vi "5.3-4.7.3-What Client.vi"() -> ()   [LabVIEW 2010]
doc: "This VI implements a client for the Named Service UDP Server.vi.\nIt connects to a service by specifying the server address and the name of the service. After sending a 'Hello' string to the server, the client receives the string sent by the server, displays the string and closes the connection.\n\n<b>Note:</b> This VI is built to work with the Named Service UDP Server.vi in UDP.llb."
uses:
  5.0-Global.vi
  <vilib>/addons/internet/NI_InternetTK_Common_VIs.lvlib
  <vilib>/Utility/tcp.llb/UDP Multicast Open.vi
  3-Midbrain/3.3-What/_typedefs/3.3.1-LIDAR Data Typedef.ctl
  4-High Neurons/4.3-What Sensor Typedef.ctl
  4-High Neurons/4.0-Timing Badass.ctl
panel:
  out "Super Heart Beat":T1
  out "data":T2
  out "Error":errorcluster
  in  "stop":bool
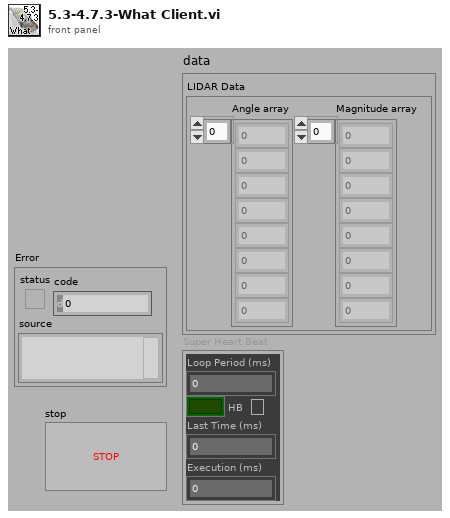
[diagram p1: front panel]
types:
  T1 = typedef "4.0-Timing Badass.ctl" = cluster{"Loop Period (ms)":u32, "HB":bool, "Last Time (ms)":u32, "Execution (ms)":u32}
  T2 = typedef "4.3-What Sensor Typedef.ctl" = cluster{"LIDAR Data":T3}
  T3 = typedef "3.3.1-LIDAR Data Typedef.ctl" = cluster{"Angle array":dbl[], "Magnitude array ":dbl[]}
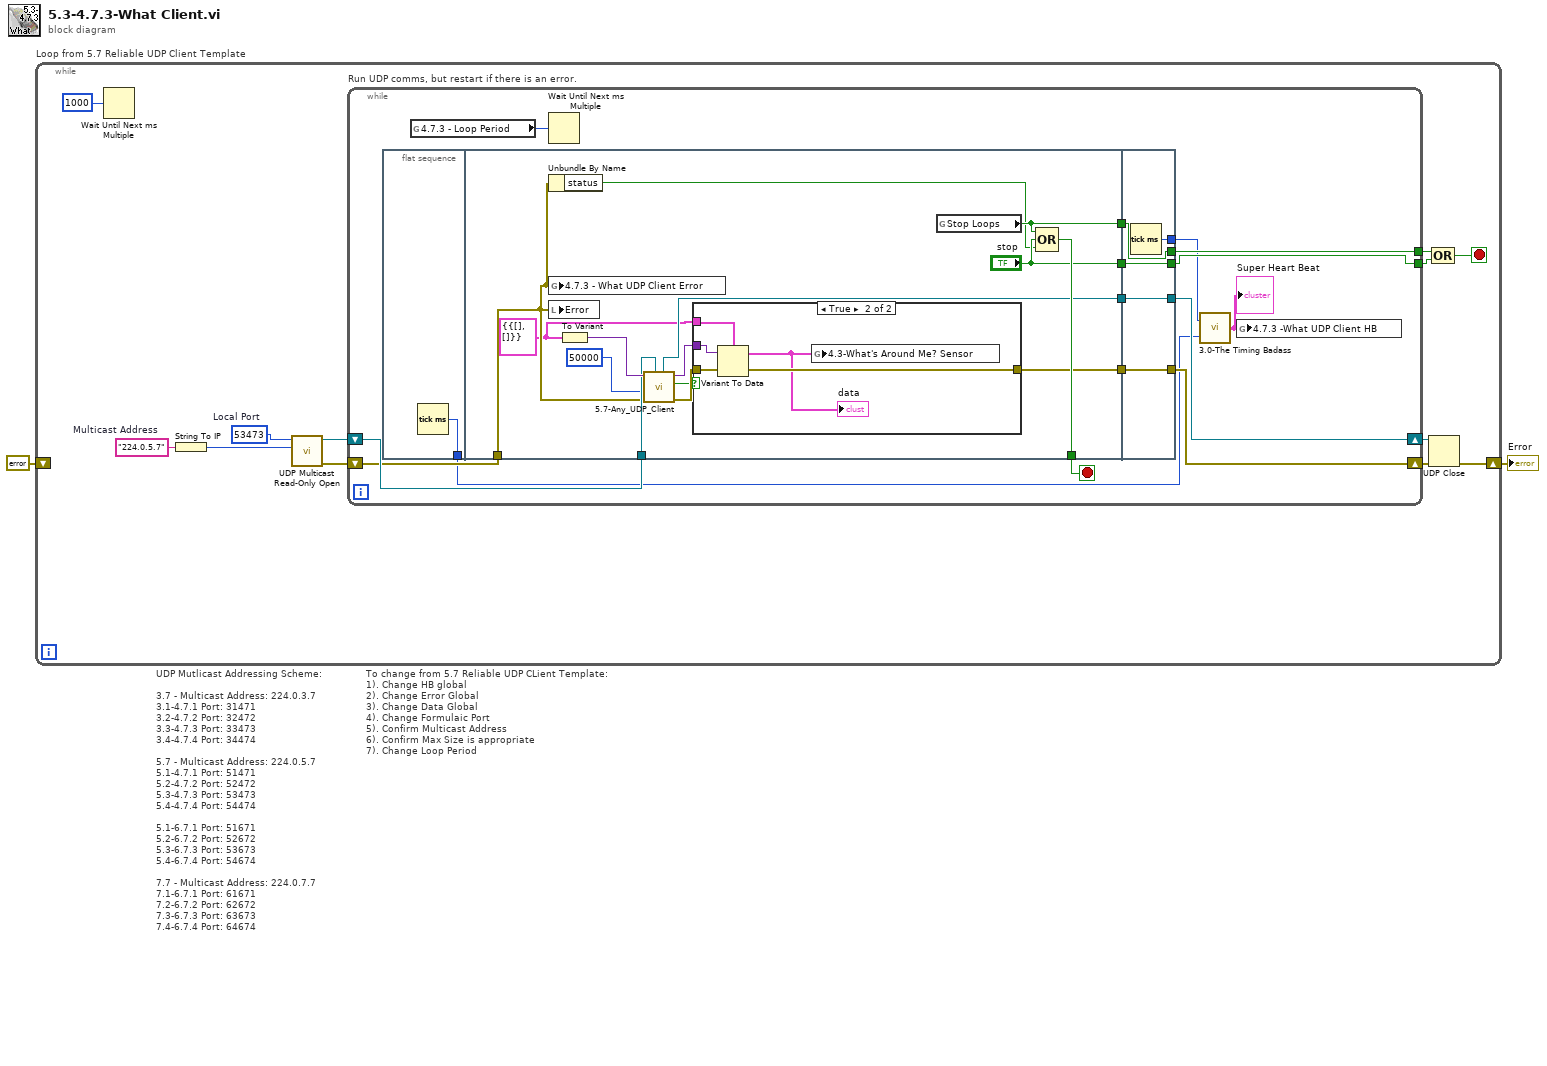
[diagram p0: block diagram]
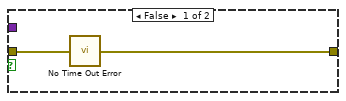
[diagram p2: hidden frame]
diagram:
  # "To change from 5.7 Reliable UDP CLient Template:\n1). Change HB global\n2). Change Error Global\n3). Change Data Global\n4). Change Formulaic Port\n5). Confirm Multicast Address\n6). Confirm Max Size is appropriate\n7). Change Loop Period"
  # "UDP Mutlicast Addressing Scheme:\n\n3.7 - Multicast Address: 224.0.3.7\n3.1-4.7.1 Port: 31471\n3.2-4.7.2 Port: 32472\n3.3-4.7.3 Port: 33473\n3.4-4.7.4 Port: 34474\n\n5.7 - Multicast Address: 224.0.5.7\n5.1-4.7.1 Port: 51471\n5.2-4.7.2 Port: 52472\n5.3-4.7.3 Port: 53473\n5.4-4.7.4 Port: 54474\n\n5.1-6.7.1 Port: 51671\n5.2-6.7.2 Port: 52672\n5.3-6.7.3 Port: 53673\n5.4-6.7.4 Port: 54674\n\n7.7 - Multicast Address: 224.0.7.7\n7.1-6.7.1 Port: 61671\n7.2-6.7.2 Port: 62672\n7.3-6.7.3 Port: 63673\n7.4-6.7.4 Port: 64674"
  n1 = while "Loop from 5.7 Reliable UDP Client Template" {
    shift-right: [w9] -> w2
    shift-left: errorcluster {"status"=FALSE, "code"=0, "source"=""} ("error out") -> [_]
    stop <- w12 stop-if-true
    w5 = u16 53473  # Local Port
    w7 = "224.0.5.7"  # Multicast Address
    n2 = Wait Until Next ms Multiple(millisecond multiple=u32 1000) -> ()  [unwired: 1 out]
    n3 = String To IP(1:w7) -> (0:w6:u32)
    n4 = call-poly <vilib>:"UDP Multicast Read-Only Open.vi"("multicast addr"=w6, "port"=w5) -> ("error out"=w3:errorcluster, "connection ID"=w4:refnum<k16>)  [unwired: 2 in, 6 out]
    n5 = while "Run UDP comms, but restart if there is an error." {
      tunnel: [w28] -> w14
      tunnel: [w27] -> w13
      shift-right: [w25] -> w11
      shift-left: w4 -> [w26]
      shift-right: [w24] -> w10
      shift-left: w3 -> [w23]
      stop <- w29 stop-if-true
      n6 = flat-sequence {
        tunnel: [w30] -> w16
        tunnel: [w44] -> w29
        tunnel: w26 -> [w38]
        tunnel: w23 -> [w33]
        tunnel: [w41] -> w21
        tunnel: ["stop"] -> w20
        tunnel: [w37] -> w19
        tunnel: [w36] -> w18
        tunnel: [w53] -> w24
        tunnel: [w54] -> w25
        tunnel: [w55] -> w27
        tunnel: [w56] -> w28
        tunnel: w21 -> [w56]
        tunnel: w20 -> [w55]
        tunnel: w19 -> [w54]
        tunnel: w18 -> [w53]
        tunnel: [w52] -> w17
        frame #0 {
          n7 = Tick Count (ms)() -> (millisecond timer value=w30:u32)
        }
        frame #1 {
          w31 = T2 {"LIDAR Data"={"Angle array"=[], "Magnitude array "=[]}} ("data")
          n8 = Unbundle By Name(w33) -> ("status"=w39:bool)
          n9 = global write "5.0-Global.vi" "4.7.3 - What UDP Client Error"(w33) -> ()
          n10 = local write "Error"(w33) -> ()
          n11 = To Variant(anything=w31) -> (Variant=w43:variant)
          n12 = call "5.7-Any_UDP_Client.vi"("Port In"=w38, "error In"=w33, "Max Size"=50000, "DataTypeIn"=w43) -> ("Error Out"=w35:errorcluster, "Check Passed"=w34:bool, "DataOut"=w42:variant, "Port out"=w37:refnum<k16>)  [unwired: 4 in]
          n13 = case "Ignore Timeouts" shown="True" w34 {
            tunnel: w42 -> [_ w51]
            tunnel: w31 -> [_ w50]
            tunnel: w35 -> [w46 w49]
            tunnel: [w45 w48] -> w36
            frame False {
              n14 = call <vilib>:"No Time Out Error.vi"("error in (no error)"=w46) -> ("error out"=w45:errorcluster)  [unwired: 14 in]
            }
            frame True {
              n15 = Variant To Data(error in=w49, Variant=w51, type=w50) -> (error out=w48:errorcluster, data=w47:T2)
              "data" <- w47
              n16 = global write "5.0-Global.vi" "4.3-What's Around Me? Sensor"(w47) -> ()
            }
          }
          n17 = global read "5.0-Global.vi" "Stop Loops"() -> (w41:bool)
          n18 = Compound Arithmetic op=OR(w41, "stop", w39) -> (w44:bool)
        }
        frame #2 {
          n19 = Tick Count (ms)() -> (millisecond timer value=w52:u32)
        }
      }
      n20 = global read "5.0-Global.vi" "4.7.3 - Loop Period"() -> (w22:u32)
      n21 = Wait Until Next ms Multiple(millisecond multiple=w22) -> ()  [unwired: 1 out]
      n22 = call "3.0-The Timing Badass.vi"("Start"=w16, "End"=w17) -> ("Super Heart Beat"=w15:T1)
      "Super Heart Beat" <- w15
      n23 = global write "5.0-Global.vi" "4.7.3 -What UDP Client HB"(w15) -> ()
    }
    n24 = UDP Close(connection ID=w11, 8:w10) -> (error out=w9:errorcluster)  [unwired: 1 out]
    n25 = Compound Arithmetic op=OR(w14, w13) -> (w12:bool)
  }
  "Error" <- w2
